vi "SetConfig.vi"(8 "error in (no error)":errorcluster, 9 "Timeout":u32, 10 "TermChr":string, 11 "OXY_SCPI Reseource In":refnum<visa-resource-name>) -> (0 "error out":errorcluster, 3 "OXY_SCPI Reseource Out":refnum<visa-resource-name>)   [LabVIEW 2020, in "OXYGEN_Datastream.lvlib"]
uses:
  OXYGEN_Datastream.lvlib
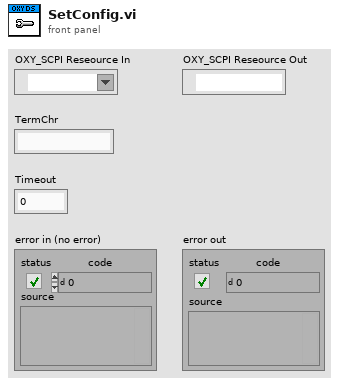
[diagram p1: front panel]
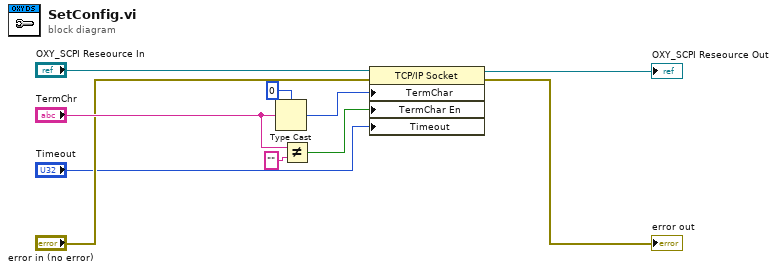
[diagram p0: block diagram]
diagram:
  n1 = Type Cast(type=u8 0 ("Message Based Settings:Termination Character"), x="TermChr") -> (*(type *) &x=w8:u8)
  n2 = Not Equal?(x="TermChr", y="") -> (x != y?=w5:bool)
  n3 = property class="TCP/IP Socket"(reference="OXY_SCPI Reseource In", error in="error in (no error)", "TermChar"=w8, "TermChar En"=w5, "Timeout"="Timeout") -> (reference out=→"OXY_SCPI Reseource Out":refnum<visa-resource-name>, error out=→"error out":errorcluster)
